vi "Read_fifo_cmd.vi"(8 "error in (no error)":errorcluster, 11 "VISA Refnum in":refnum<visa-resource-name>) -> (0 "error out":errorcluster, 1 "Data_out":u8[](array[numeric]), 2 "Bytes":u32, 3 "VISA Refnum out":refnum<visa-resource-name>)   [LabVIEW 2019]
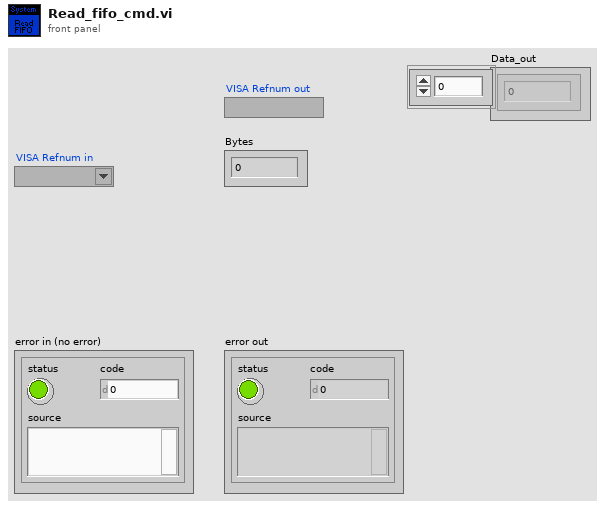
[diagram p1: front panel]
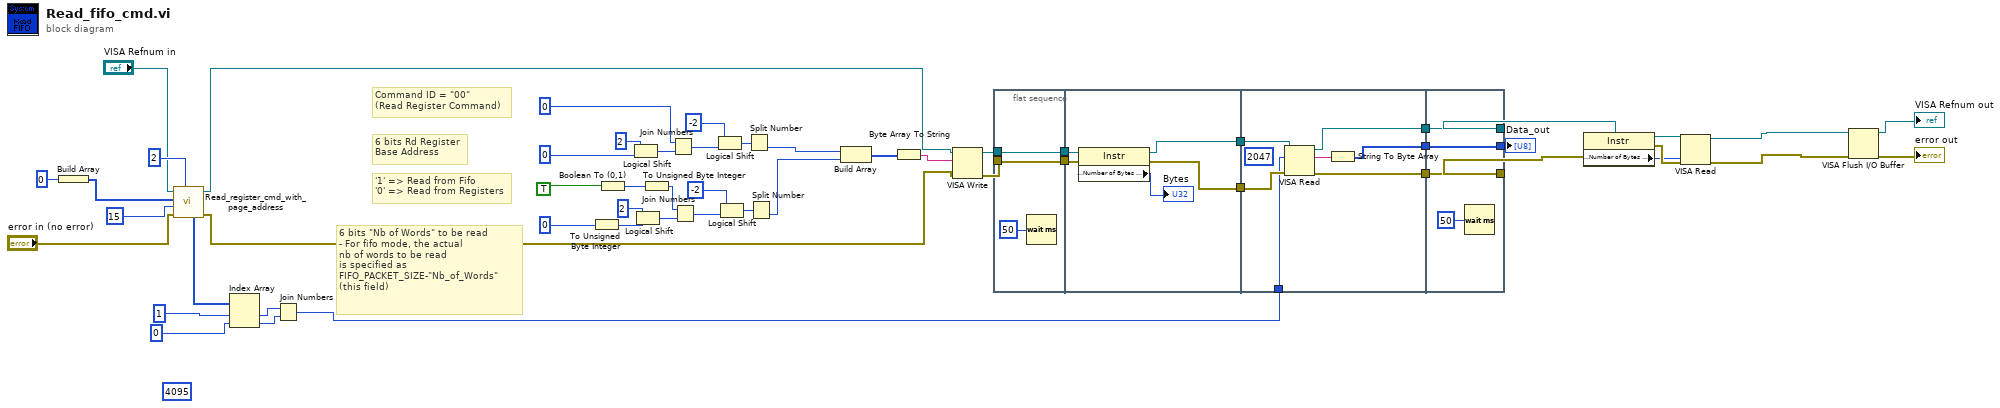
[diagram p0: block diagram]
diagram:
  (unwired) 4095 ("index")
  # "'1' => Read from Fifo\n'0' => Read from Registers"
  # "6 bits \"Nb of Words\" to be read\n- For fifo mode, the actual \nnb of words to be read \nis specified as \nFIFO_PACKET_SIZE-\"Nb_of_Words\" \n(this field)"
  # "6 bits Rd Register \nBase Address"
  # "Command ID = \"00\" \n(Read Register Command)"
  n1 = Build Array(u8 0 ("element")) -> (w23:u8[])
  n2 = call "Read_register_cmd_with_page_address.vi"("Words_to_read"=u16 2, "error in (no error)"="error in (no error)", "Register Address"=u8 15, "Page address"=w23, "VISA Refnum in"="VISA Refnum in") -> ("error out"=w19:errorcluster, "VISA Refnum out"=w21:refnum<visa-resource-name>, "RdReg Data"=w18:u8[])  [unwired: 4 in]
  n3 = Index Array(array=w18, index #1=1 ("index"), index #2=0 ("index")) -> (element #1=w16:u8, element #2=w15:u8)
  n4 = Join Numbers(hi=w16, lo=w15) -> ((hi.lo)=w13:u16)
  n5 = To Unsigned Byte Integer(number=u8 0 ("t")) -> (unsigned 8bit integer=w35:u8)
  n6 = Boolean To (0,1)(Boolean=TRUE ("Fifo-mode En")) -> (0, 1=w39:i16)
  n7 = Logical Shift(y=i16 2, x=u8 0 ("RdReg Addr")) -> (x << y=w50:u8)
  n8 = Logical Shift(y=i16 2, x=w35) -> (x << y=w43:u8)
  n9 = To Unsigned Byte Integer(number=w39) -> (unsigned 8bit integer=w38:u8)
  n10 = Join Numbers(hi=u8 0, lo=w50) -> ((hi.lo)=w51:u16)
  n11 = Join Numbers(hi=w38, lo=w43) -> ((hi.lo)=w42:u16)
  n12 = Logical Shift(y=i16 -2, x=w51) -> (x << y=w47:u16)
  n13 = Logical Shift(y=i16 -2, x=w42) -> (x << y=w45:u16)
  n14 = Split Number(x=w47) -> (lo(x)=w46:u8)  [unwired: 1 out]
  n15 = Split Number(x=w45) -> (lo(x)=w40:u8)  [unwired: 1 out]
  n16 = Build Array(w46, w40) -> (w36:u8[])
  n17 = Byte Array To String(unsigned byte array=w36) -> (string=w37:string)
  n18 = VISA Write(VISA resource name=w21, write buffer=w37, error in (no error)=w19) -> (VISA resource name out=w30:refnum<visa-resource-name>, error out=w31:errorcluster)  [unwired: 1 out]
  n19 = flat-sequence {
    tunnel: w30 -> [w56]
    tunnel: w31 -> [w57]
    tunnel: [w57] -> w32
    tunnel: [w56] -> w33
    tunnel: w33 -> [w61]
    tunnel: w32 -> [w62]
    tunnel: [w59] -> w29
    tunnel: [w58] -> w28
    tunnel: w29 -> [w68]
    tunnel: w28 -> [w67]
    tunnel: w13 -> [w63]
    tunnel: [w65] -> w8
    tunnel: [w66] -> w7
    tunnel: [w64] -> w6
    tunnel: [w71] -> w27
    tunnel: [w72] -> w11
    tunnel: [w73] -> w12
    tunnel: w8 -> [w73]
    tunnel: w7 -> [w72]
    tunnel: w6 -> [w71]
    frame #0 {
      n20 = Wait (ms)(milliseconds to wait=u32 50) -> ()  [unwired: 1 out]
    }
    frame #1 {
      n21 = property class="Instr"(reference=w61, error in=w62) -> (reference out=w58:refnum<visa-resource-name>, error out=w59:errorcluster, "Serial Settings:Number of Bytes at Serial Port"=→"Bytes":u32)
    }
    frame #2 {
      (unwired) u32 2047 ("byte count")
      n22 = VISA Read(VISA resource name=w67, byte count=w63, error in (no error)=w68) -> (VISA resource name out=w65:refnum<visa-resource-name>, read buffer=w69:string, error out=w66:errorcluster)  [unwired: 1 out]
      n23 = String To Byte Array(string=w69) -> (unsigned byte array=w64:u8[])
    }
    frame #3 {
      n24 = Wait (ms)(milliseconds to wait=u32 50) -> ()  [unwired: 1 out]
    }
  }
  n25 = property class="Instr"(reference=w12, error in=w11) -> (reference out=w5:refnum<visa-resource-name>, error out=w4:errorcluster, "Serial Settings:Number of Bytes at Serial Port"=w3:u32)
  n26 = VISA Read(VISA resource name=w5, byte count=w3, error in (no error)=w4) -> (VISA resource name out=w1:refnum<visa-resource-name>, error out=w2:errorcluster)  [unwired: 2 out]
  n27 = VISA Flush I/O Buffer(VISA resource name=w1, error in (no error)=w2) -> (VISA resource name out=→"VISA Refnum out":refnum<visa-resource-name>, error out=→"error out":errorcluster)  [unwired: 1 in]
  "Data_out" <- w27
